vi "CMR.vi"() -> ()   [LabVIEW 2016]
uses:
  <vilib>/Math Plots/2D Math Plots/2D Compass/2D Compass XCtrl/2D Compass.xctl
  <vilib>/Math Plots/2D Math Plots/2D Compass/2D Compass Datatype/2D Compass Datatype.lvclass
  <vilib>/Math Plots/2D Math Plots/2D Compass/2D Compass Datatype/Public/Plot Helper (Vector).vi
panel:
  out "CMR y":dbl=-1.4999999999999996
  out "CMR x":dbl=-3.885780586188048e-16
  out "A. vector res.":dbl=270.0
  out "M. vector res.":dbl=1.4999999999999996
  out "M. vector 240°":dbl=0.8660254037844384
  out "M. vector 120°":dbl=0.8660254037844387
  out "M. vector 0°":dbl
  in  "Detener":bool
  in  "Frecuencia":dbl=1.0
  out "Campo margnético rotativo":refnum<class "2D Plot Datatype.lvclass">[](xcontrol) caption="2D Compass"
  # "B"
  # "M"
  # "B"
  # "M"
  # "B"
  # "M"
  # "B"
  # "M"
  # "°"
  # "Luis Alberto López Durán"
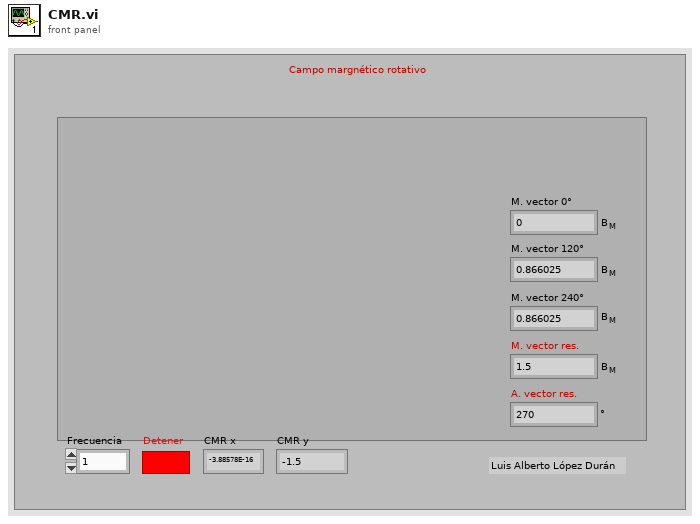
[diagram p1: front panel]
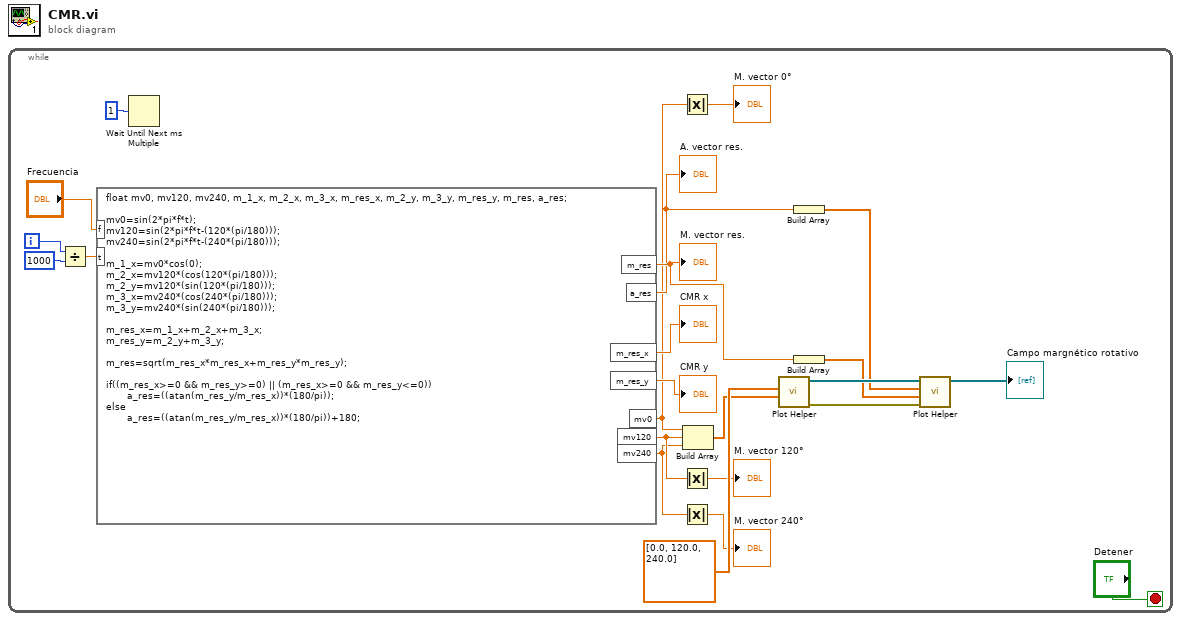
[diagram p0: block diagram]
diagram:
  n1 = while {
    i -> [w7]
    stop <- "Detener" stop-if-true
    n2 = Divide(x=w7, y=1000) -> (x/y=w4:dbl)
    n3 = formula code="float mv0, mv120, mv240, m_1_x, m_2_x, m_3_x, m_res_x, m_2_y, m_3_y, m_res_y, m_res, a_res;\n\nmv0=sin(2*pi*f*t);\nmv120=sin(2*pi*f*t-(120*(pi/180)));\nmv240=sin(2*pi*f*t-(240*(pi/180)));\n\nm_1_x=mv0*cos(0);\nm_2_x=mv120*(cos(120*(pi/180)));\nm_2_y=mv120*(sin(120*(pi/180)));\nm_3_x=mv240*(cos(240*(pi/180)));\nm_3_y=mv240*(sin(240*(pi/180)));\n\nm_res_x=m_1_x+m_2_x+m_3_x;\nm_res_y=m_2_y+m_3_y;\n\nm_res=sqrt(m_res_x*m_res_x+m_res_y*m_res_y);\n\nif((m_res_x>=0 && m_res_y>=0) || (m_res_x>=0 && m_res_y<=0))\n       a_res=((atan(m_res_y/m_res_x))*(180/pi));\nelse\n       a_res=((atan(m_res_y/m_res_x))*(180/pi))+180;"("f"="Frecuencia", "t"=w4) -> ("m_res"=w16:dbl, "a_res"=w13:dbl, "m_res_x"=→"CMR x":dbl, "m_res_y"=→"CMR y":dbl, "mv0"=w3:dbl, "mv120"=w2:dbl, "mv240"=w1:dbl)
    "M. vector res." <- w16
    "A. vector res." <- w13
    n4 = Wait Until Next ms Multiple(millisecond multiple=u32 1) -> ()  [unwired: 1 out]
    n5 = Absolute Value(x=w3) -> (abs(x)=→"M. vector 0°":dbl)
    n6 = Absolute Value(x=w2) -> (abs(x)=→"M. vector 120°":dbl)
    n7 = Absolute Value(x=w1) -> (abs(x)=→"M. vector 240°":dbl)
    n8 = Build Array(w3, w2, w1) -> (w20:dbl[])
    n9 = call-poly <vilib>:"Plot Helper.vi"("radius vector"=w20, "theta vector"=dbl[] [0.0, 120.0, 240.0]) -> ("error out"=w18:errorcluster, "2D Plot Class Obj Array out"=w19:refnum<class "2D Plot Datatype.lvclass">[])  [unwired: 2 in, 6 out]
    n10 = Build Array(w13) -> (w17:dbl[])
    n11 = Build Array(w16) -> (w15:dbl[])
    n12 = call-poly <vilib>:"Plot Helper.vi"("error in (no error)"=w18, "radius vector"=w15, "theta vector"=w17, "2D Plot Class Obj Array in"=w19) -> ("2D Plot Class Obj Array out"=→"Campo margnético rotativo":refnum<class "2D Plot Datatype.lvclass">[])  [unwired: 7 out]
  }
